vi "RefTest2.vi"(10 "String":string, 11 "String in":refnum<vi>) -> ()   [LabVIEW 2014]
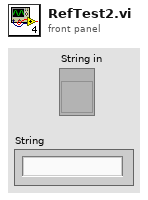
[diagram p1: front panel]
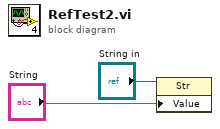
[diagram p0: block diagram]
diagram:
  n1 = property on="Property Node" class="Str"(reference="String in", "Value"="String") -> ()  [unwired: 1 in, 2 out]
